vi "End LabviewIngestService IngestDataStreamString.vi"(8 "error in":errorcluster, 11 "Call ID in":T3) -> (0 "error out":errorcluster, 1 "errorDetails":T1, 2 "Response Data":T2)   [LabVIEW 2024, in "SiftProxy_client.lvlib"]
uses:
  SiftProxy_client.lvlib
  <vilib>/gRPC/LabVIEW gRPC Library/Shared/grpcId.ctl
  RPC Messages/sift_proxy_v1_IngestDataStreamResponse.ctl
  <vilib>/gRPC/LabVIEW gRPC Library/Shared/Any.ctl
  RPC Messages/sift_proxy_v1_IngestDataStreamResponse_Flat.ctl
  2435b599-b0f7-48e4-804e-62ee509d3e35.vi
  <vilib>/gRPC/LabVIEW gRPC Library/Shared/TranslateGrpcError.vi
  <vilib>/gRPC/LabVIEW gRPC Library/Shared/Wait On Occurrence Wrapper.vi
  <vilib>/gRPC/LabVIEW gRPC Library/Shared/Wait On Occurence.vi
  <vilib>/gRPC/LabVIEW gRPC Library/Server API/Server/Get Server DLL Path.vi
  <vilib>/Utility/error.llb/Error Cluster From Error Code.vi
  <vilib>/Utility/config.llb/Open Config Data.vi
  <vilib>/Utility/config.llb/Write Key.vi
  <vilib>/Utility/config.llb/Write Key (Boolean).vi
  <vilib>/Utility/config.llb/Not A Config Data Refnum.vi
  <vilib>/Utility/config.llb/Read Key.vi
  <vilib>/Utility/config.llb/Read Key (Boolean).vi
  <vilib>/Utility/config.llb/Close Config Data.vi
  <vilib>/gRPC/LabVIEW gRPC Library/grpc-lvsupport-release.lvlib
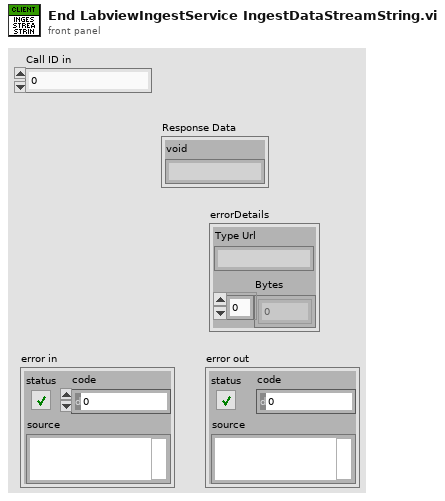
[diagram p1: front panel]
types:
  T1 = typedef "grpc-lvsupport-release.lvlib/Any.ctl" = cluster{"Type Url":string, "Bytes":u8[]}
  T2 = typedef "SiftProxy_client.lvlib/sift_proxy_v1_IngestDataStreamResponse.ctl" = cluster{"void":string}
  T3 = typedef "grpc-lvsupport-release.lvlib/grpcId.ctl" = u64
  T4 = typedef "SiftProxy_client.lvlib/sift_proxy_v1_IngestDataStreamResponse_Flat.ctl" = cluster{"void":string}
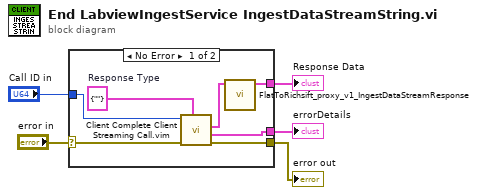
[diagram p0: block diagram]
diagram:
  n1 = case shown="No Error" "error in" {
    selector: "error in" -> [w12 w13]
    tunnel: [w11 w13] -> w4
    tunnel: "Call ID in" -> [w10 _]
    tunnel: [w6 _] -> w2
    tunnel: [w8 _] -> w1
    frame No Error {
      w9 = T4 {"void"=""}  # Response Type
      n2 = call "Client Complete Client Streaming Call.vim"("Response Type"=w9, "error in"=w12, "Call ID in"=w10) -> ("error out"=w11:errorcluster, "errorDetails"=w8:T1, "Response Data"=w7:T4)  [unwired: 6 in]
      n3 = call "FlatToRichsift_proxy_v1_IngestDataStreamResponse.vi"("InputCluster"=w7) -> ("OutputCluster"=w6:T2)  [unwired: 10 in]
    }
    frame Error {
    }
  }
  "error out" <- w4
  "Response Data" <- w2
  "errorDetails" <- w1
